vi "AggregationRate_Set.vi"(8 "error in (no error)":errorcluster, 10 "Aggregation Rate (s) (<0 for NONE)":dbl, 11 "OXY_SCPI Reseource In":refnum<visa-resource-name>) -> (0 "error out":errorcluster, 1 "communication_data":T1, 3 "OXY_SCPI Reseource Out":refnum<visa-resource-name>)   [LabVIEW 2018, in "OXYGEN.lvlib"]
doc: "Set numeric data aggregation time for output."
uses:
  OXYGEN.lvlib
  TypeDefs/Cluster_RawCommData.ctl
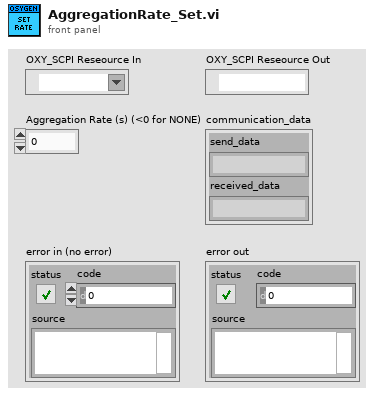
[diagram p1: front panel]
types:
  T1 = typedef "OXYGEN.lvlib/Cluster_RawCommData.ctl" = cluster{"send_data":string, "received_data":string}
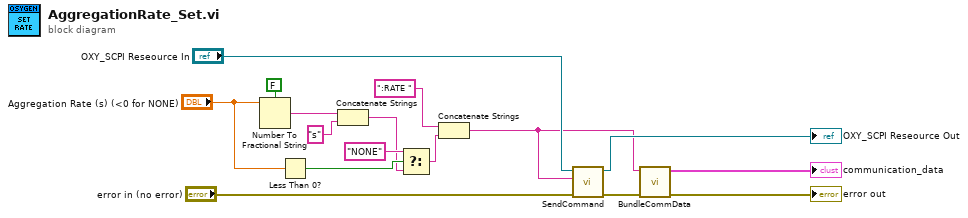
[diagram p0: block diagram]
diagram:
  n1 = Number To Fractional String(use system decimal point (T)=FALSE, number="Aggregation Rate (s) (<0 for NONE)") -> (F-format string=w3:string)  [unwired: 2 in]
  n2 = Less Than 0?(x="Aggregation Rate (s) (<0 for NONE)") -> (x < 0?=w7:bool)
  n3 = Concatenate Strings(w3, "s" ("string")) -> (w1:string)
  n4 = Select(t="NONE", s=w7, f=w1) -> (s? t:f=w5:string)
  n5 = Concatenate Strings(":RATE " ("string"), w5) -> (w10:string)
  n6 = call "SendCommand.vi"("error in (no error)"="error in (no error)", "String to Send"=w10, "OXY_SCPI Reseource In"="OXY_SCPI Reseource In") -> ("error out"=w11:errorcluster, "OXY_SCPI Reseource Out"=→"OXY_SCPI Reseource Out":refnum<visa-resource-name>)  [unwired: 7 in]
  n7 = call "BundleCommData.vi"("error in (no error)"=w11, "send_data"=w10) -> ("error out"=→"error out":errorcluster, "communication_data"=→"communication_data":T1)  [unwired: 8 in]
